vi "等间隔时刻（时分秒）闹钟.vi"(8 "Error In":errorcluster caption="错误输入", 9 "模式":enum16{"秒", "分", "时"}(ring), 10 "间隔":u32) -> (0 "Error Out":errorcluster caption="错误输出", 1 "时刻":i32, 3 "时间到":bool)   [LabVIEW 2012]
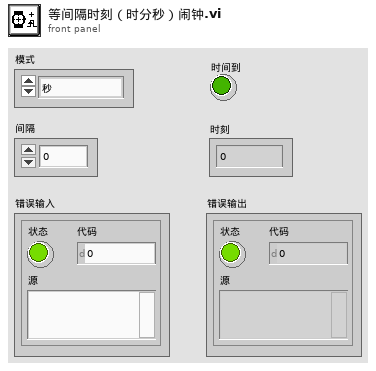
[diagram p1: front panel]
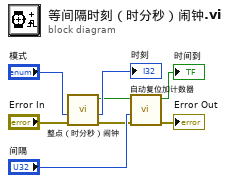
[diagram p0: block diagram]
diagram:
  n1 = call "整点（时分秒）闹钟.vi"("Error In"="Error In", "模式"="模式") -> ("Error Out"=w3:errorcluster, "时刻"=→"时刻":i32, "时间到"=w4:bool)  [unwired: 7 in]
  n2 = call "自动复位加计数器.vi"("error in"=w3, "preset value"="间隔", "count up"=w4) -> ("error out"=→"Error Out":errorcluster, "done"=→"时间到":bool)  [unwired: 6 in, 1 out]
